vi "Read ArgumentDefault.vi"(8 "error in (no error)":errorcluster, 11 "ArgumentParser in":refnum<class "ArgumentParser.lvclass">) -> (0 "error out":errorcluster, 2 "ArgumentDefault":string, 3 "ArgumentParser out":refnum<class "ArgumentParser.lvclass">)   [LabVIEW 2022 SP3, in "ArgumentParser.lvlib" / "ArgumentParser.lvclass"]
uses:
  ArgumentParser.lvclass
  ArgumentParser.lvclass/ArgumentParser.ctl
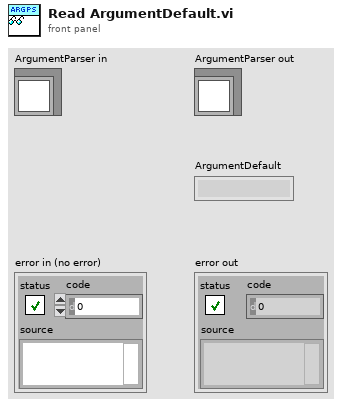
[diagram p1: front panel]
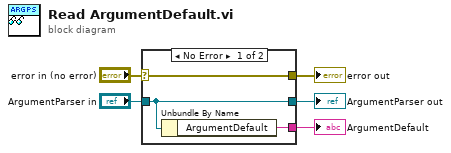
[diagram p0: block diagram]
diagram:
  n1 = case shown="No Error" "error in (no error)" {
    selector: "error in (no error)" -> [w8 w9]
    tunnel: [w8 w9] -> w4
    tunnel: [w7 w10] -> w2
    tunnel: "ArgumentParser in" -> [w7 w10]
    tunnel: [w6 _] -> w1
    frame No Error {
      n2 = Unbundle By Name(w7) -> ("ArgumentDefault"=w6:string)
    }
    frame Error {
    }
  }
  "error out" <- w4
  "ArgumentParser out" <- w2
  "ArgumentDefault" <- w1
